vi "ExplanationToError.vi"(9 "Explanation in":string) -> (1 "Error out":errorcluster)   [LabVIEW 2017, in "GPError.lvlib"]
doc: "Decodes <B>Explanation in</B> and creates an error cluster returned in <B>Error out</B> from that string.\n\nThis VI is localized to English language.\n\nThis VI is inlined.\n\nSteen Schmidt\nGPower\n11/7 2013"
uses:
  GPError.lvlib
panel:
  # "Copyright © 2013\nSteen Schmidt, GPower\nSee enclosed license file for terms and conditions"
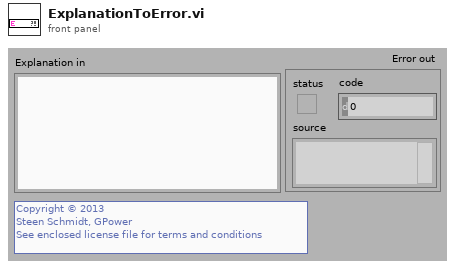
[diagram p1: front panel]
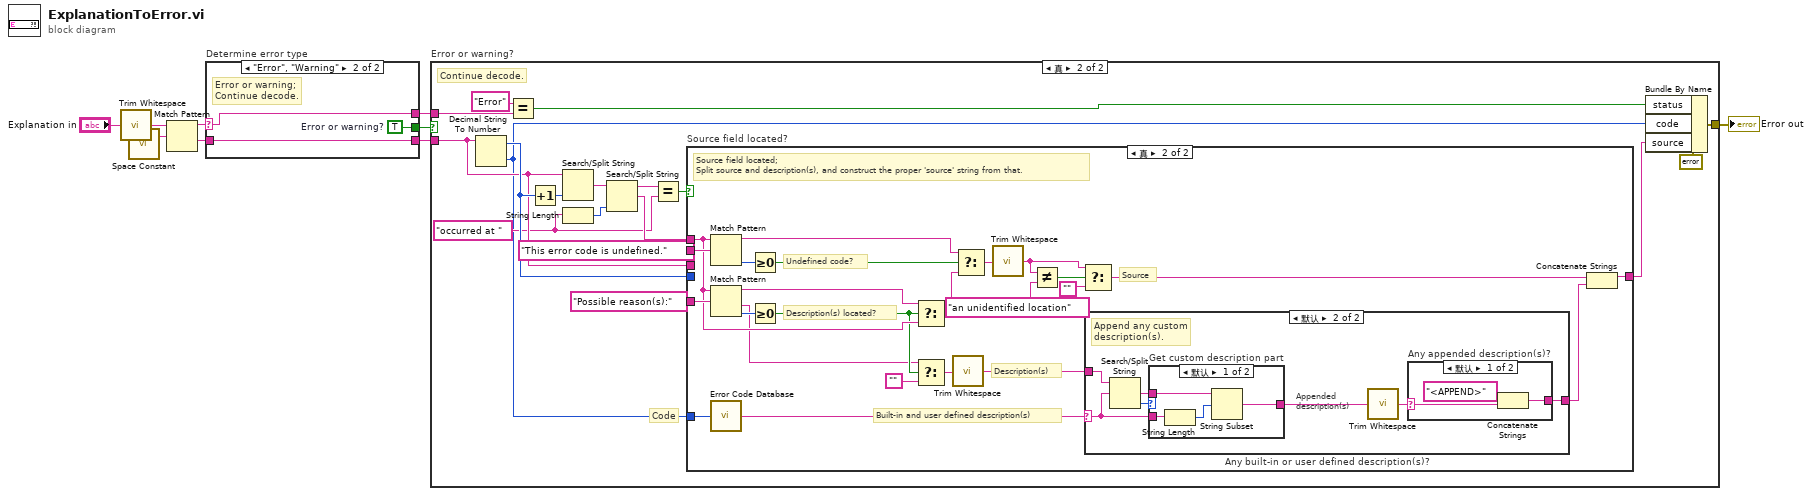
[diagram p0: block diagram]
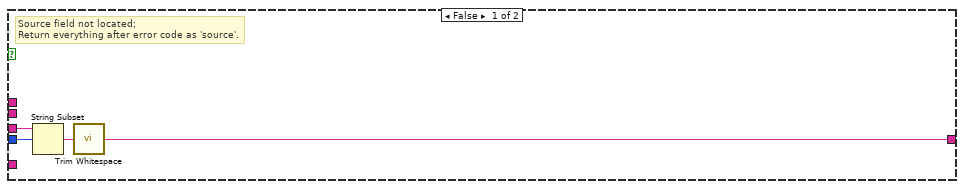
[diagram p3: hidden frame]
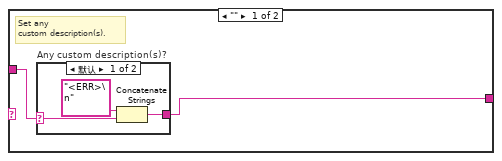
[diagram p4: hidden frame]
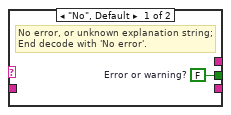
[diagram p8: hidden frame]
diagram:
  n1 = call <vilib>:"Trim Whitespace.vi"("string"="Explanation in") -> ("trimmed string"=w8:string)  [unwired: 1 in]
  n2 = call <vilib>:"Space Constant.vi"() -> ("String"=w7:string)
  n3 = Match Pattern(string=w8, regular expression=w7) -> (before substring=w6:string, after substring=w5:string)  [unwired: 1 in, 2 out]
  n4 = case "Determine error type" shown="\"Error\", \"Warning\"" w6 {
    selector: w6 -> [_ w11]
    tunnel: w5 -> [_ w13]
    tunnel: [_ w13] -> w3
    tunnel: [w10 w12] -> w4
    tunnel: [_ w11] -> w2
    frame "No", Default {
      w10 = FALSE  # Error or warning?
      # "No error, or unknown explanation string;\nEnd decode with 'No error'."
    }
    frame "Error", "Warning" {
      w12 = TRUE  # Error or warning?
      # "Error or warning;\nContinue decode."
    }
  }
  n5 = case "Error or warning?" shown="真" w4 {
    tunnel: w3 -> [_ w22]
    tunnel: w2 -> [_ w31]
    tunnel: [_ w27] -> w1
    frame False {
      # "End decode with 'No error'."
    }
    frame True {
      w16 = "occurred at "
      # "Code"
      # "Continue decode."
      n6 = Decimal String To Number(string=w22) -> (offset past number=w26:i32, number=w14:i32)  [unwired: 2 in]
      n7 = Equal?(x="Error", y=w31) -> (x = y?=w28:bool)
      n8 = Increment(x=w26) -> (x+1=w21:i32)
      n9 = Search/Split String(string=w22, offset (0)=w21) -> (match + rest of string=w20:string)  [unwired: 1 in, 2 out]
      n10 = String Length(string=w16) -> (length=w19:i32)
      n11 = Search/Split String(string=w20, offset (0)=w19) -> (substring before match=w18:string, match + rest of string=w17:string)  [unwired: 1 in, 1 out]
      n12 = Equal?(x=w18, y=w16) -> (x = y?=w15:bool)
      n13 = case "Source field located?" shown="真" w15 {
        tunnel: w22 -> [w35 _]
        tunnel: w26 -> [w34 _]
        tunnel: [w32 w38] -> w25
        tunnel: "This error code is undefined." -> [_ w59]
        tunnel: w17 -> [_ w52]
        tunnel: "Possible reason(s):" -> [_ w58]
        tunnel: w14 -> [_ w41]
        frame False {
          # "Source field not located;\nReturn everything after error code as 'source'."
          n14 = String Subset(string=w35, offset (0)=w34) -> (substring=w33:string)  [unwired: 1 in]
          n15 = call <vilib>:"Trim Whitespace.vi"("string"=w33) -> ("trimmed string"=w32:string)  [unwired: 1 in]
        }
        frame True {
          # "Built-in and user defined description(s)"
          # "Description(s)"
          # "Description(s) located?"
          # "Source"
          # "Undefined code?"
          # "Source field located;\nSplit source and description(s), and construct the proper 'source' string from that."
          n16 = Match Pattern(string=w52, regular expression=w59) -> (before substring=w55:string, offset past match=w57:i32)  [unwired: 1 in, 2 out]
          n17 = Match Pattern(string=w52, regular expression=w58) -> (before substring=w53:string, after substring=w44:string, offset past match=w54:i32)  [unwired: 1 in, 1 out]
          n18 = call <vilib>:"Error Code Database.vi"("Error Code"=w41) -> ("Error Text"=w37:string)
          n19 = Greater Or Equal To 0?(x=w57) -> (x >= 0?=w56:bool)
          n20 = Greater Or Equal To 0?(x=w54) -> (x >= 0?=w45:bool)
          n21 = Select(t=w53, s=w45, f=w52) -> (s? t:f=w51:string)
          n22 = Select(t=w44, s=w45, f="") -> (s? t:f=w42:string)
          n23 = call <vilib>:"Trim Whitespace.vi"("string"=w42) -> ("trimmed string"=w40:string)  [unwired: 1 in]
          n24 = Select(t=w55, s=w56, f=w51) -> (s? t:f=w50:string)
          n25 = call <vilib>:"Trim Whitespace.vi"("string"=w50) -> ("trimmed string"=w47:string)  [unwired: 1 in]
          n26 = Not Equal?(x=w47, y="an unidentified location") -> (x != y?=w48:bool)
          n27 = Select(t=w47, s=w48, f="") -> (s? t:f=w39:string)
          n28 = case "Any built-in or user defined description(s)?" shown="默认" w37 {
            selector: w37 -> [_ w65]
            tunnel: w40 -> [w61 w67]
            tunnel: [w60 w70] -> w36
            frame "" {
              # "Set any\ncustom description(s)."
              n29 = case "Any custom description(s)?" shown="默认" w61 {
                selector: w61 -> [w64 _]
                tunnel: [w62 _] -> w60
                frame Default {
                  n30 = Concatenate Strings("<ERR>\n", w64) -> (w62:string)
                }
                frame "" {
                }
              }
            }
            frame Default {
              # "Append any custom\ndescription(s)."
              # "Appended\ndescription(s)"
              n31 = Search/Split String(string=w67, search string/char (-)=w65) -> (match + rest of string=w68:string, offset of match=w69:i32)  [unwired: 1 in, 1 out]
              n32 = case "Get custom description part" shown="默认" w69 {
                tunnel: w68 -> [w74 _]
                tunnel: w65 -> [w75 _]
                tunnel: [w72 _] -> w66
                frame Default {
                  n33 = String Length(string=w75) -> (length=w73:i32)
                  n34 = String Subset(string=w74, offset (0)=w73) -> (substring=w72:string)  [unwired: 1 in]
                }
                frame -1 {
                }
              }
              n35 = call <vilib>:"Trim Whitespace.vi"("string"=w66) -> ("trimmed string"=w71:string)  [unwired: 1 in]
              n36 = case "Any appended description(s)?" shown="默认" w71 {
                selector: w71 -> [w78 _]
                tunnel: [w76 _] -> w70
                frame Default {
                  n37 = Concatenate Strings("<APPEND>", w78) -> (w76:string)
                }
                frame "" {
                }
              }
            }
          }
          n38 = Concatenate Strings(w39, w36) -> (w38:string)
        }
      }
      n39 = Bundle By Name(cluster=errorcluster {"status"=FALSE, "code"=0, "source"=""} ("error out"), "status"=w28, "code"=w14, "source"=w25) -> (w27:errorcluster)
    }
  }
  "Error out" <- w1
